vi "LDF Get Master Name.vi"(10 "pMasterName":string, 11 "LDFHandle":u64) -> (2 "pMasterName out":string, 3 "function return":i32)   [LabVIEW 2010, in "ldf_parser.lvlib"]
doc: "int WINAPI LDF_GetMasterName(long long LDFHandle, char* pMasterName);"
uses:
  ldf_parser.lvlib
  USB2XXX/trunk/USB2XXX/USB2XXX/vs2019/Release/USB2XXX.dll
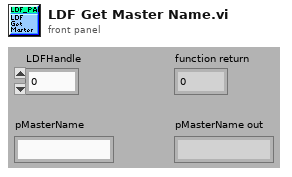
[diagram p1: front panel]
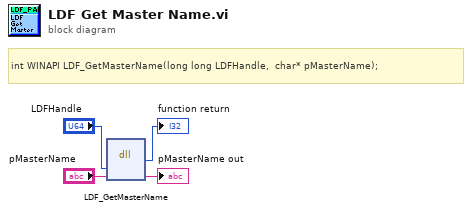
[diagram p0: block diagram]
diagram:
  # "int WINAPI LDF_GetMasterName(long long LDFHandle,  char* pMasterName);"
  n1 = dll-call lib="E:/Projects/USB2XXX/trunk/USB2XXX/USB2XXX/vs2019/Release/USB2XXX.*" fn="LDF_GetMasterName"("LDFHandle"="LDFHandle", "pMasterName"="pMasterName") -> (→"function return":i32, "pMasterName"=→"pMasterName out":string)  [unwired: 4 in, 2 out]
